vi "Graphics Folder.vi"() -> (1 "Graphics Folder":path)   [LabVIEW 2020, in "VolatusGUIControls.lvlib"]
uses:
  VolatusGUIControls.lvlib
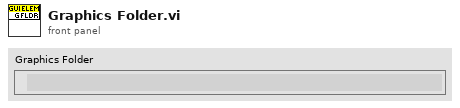
[diagram p1: front panel]
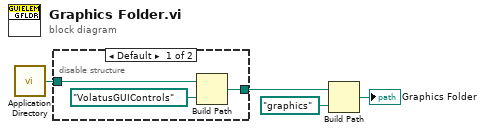
[diagram p0: block diagram]
diagram:
  n1 = call <vilib>:"Application Directory.vi"() -> ("Application Directory"=w4:path)
  n2 = disable-structure shown="Default" {
    disable-tunnel: w4 -> [w7 w8]
    disable-tunnel: [w5 w8] -> w2
    frame condition #0 (active) {
      n3 = Build Path(base path=w7, name or relative path=path "VolatusGUIControls") -> (appended path=w5:path)
    }
    frame condition #1 {
    }
  }
  n4 = Build Path(base path=w2, name or relative path=path "graphics") -> (appended path=→"Graphics Folder":path)
